vi "Test_communication_XL80.vi"() -> ()   [LabVIEW 2019]
uses:
  Library/Class/Renishaw-XL80/Renishaw-XL80.lvclass
panel:
  out "GetLaserMeasurement":dbl
  out "pStatus":i32(ring) items=["COUNT_OK"=0, "COUNT_ERROR"=1, "COUNT_TPIN_OCCURRED"=2, "COUNT_DATUMED"=4]
  out "Renishaw-XL80 out":refnum<class "Renishaw-XL80.lvclass">
  out "error out":errorcluster
  out "Connect":bool
  out "Serial Number":string
  in  "error in (no error)":errorcluster
  out "Signal Strength":i16
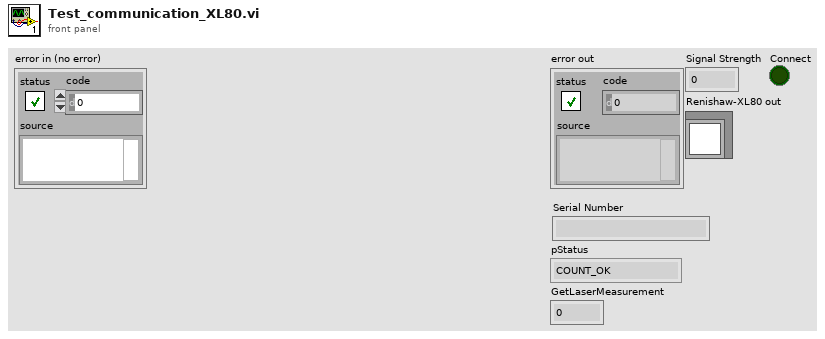
[diagram p1: front panel]
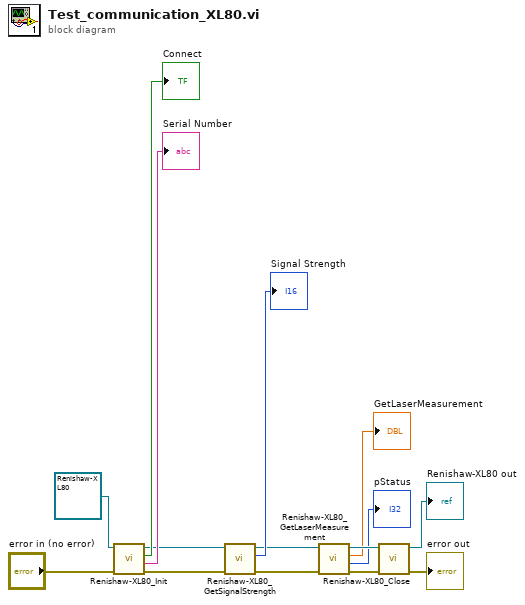
[diagram p0: block diagram]
diagram:
  n1 = call-dynamic "Renishaw-XL80_Init.vi"("error in (no error)"="error in (no error)", "Renishaw-XL80 in"=refnum<class "Renishaw-XL80.lvclass"> refnum ("Renishaw-XL80.lvclass")) -> ("error out"=w3:errorcluster, "Serial Number"=→"Serial Number":string, "Connect"=→"Connect":bool, "Renishaw-XL80 out"=w4:refnum<class "Renishaw-XL80.lvclass">)  [unwired: 6 in]
  n2 = call-dynamic "Renishaw-XL80_GetSignalStrength.vi"("error in (no error)"=w3, "Renishaw-XL80 in"=w4) -> ("error out"=w1:errorcluster, "Signal Strength"=→"Signal Strength":i16, "Renishaw-XL80 out"=w2:refnum<class "Renishaw-XL80.lvclass">)  [unwired: 7 in]
  n3 = call-dynamic "Renishaw-XL80_GetLaserMeasurement.vi"("error in (no error)"=w1, "Renishaw-XL80 in"=w2) -> ("error out"=w9:errorcluster, "pStatus"=→"pStatus":i32, "GetLaserMeasurement"=→"GetLaserMeasurement":dbl, "Renishaw-XL80 out"=w10:refnum<class "Renishaw-XL80.lvclass">)  [unwired: 6 in]
  n4 = call-dynamic "Renishaw-XL80_Close.vi"("error in (no error)"=w9, "Renishaw-XL80 in"=w10) -> ("error out"=→"error out":errorcluster, "Renishaw-XL80 out"=→"Renishaw-XL80 out":refnum<class "Renishaw-XL80.lvclass">)  [unwired: 8 in]
